vi "write_environment.vi"(9 "Expression":T1, 10 "symbol":string, 11 "Environment in":T3) -> (3 "Environment out":T3)   [LabVIEW 2020]
uses:
  ExpressionType.ctl
  Expression.ctl
  Environment.ctl
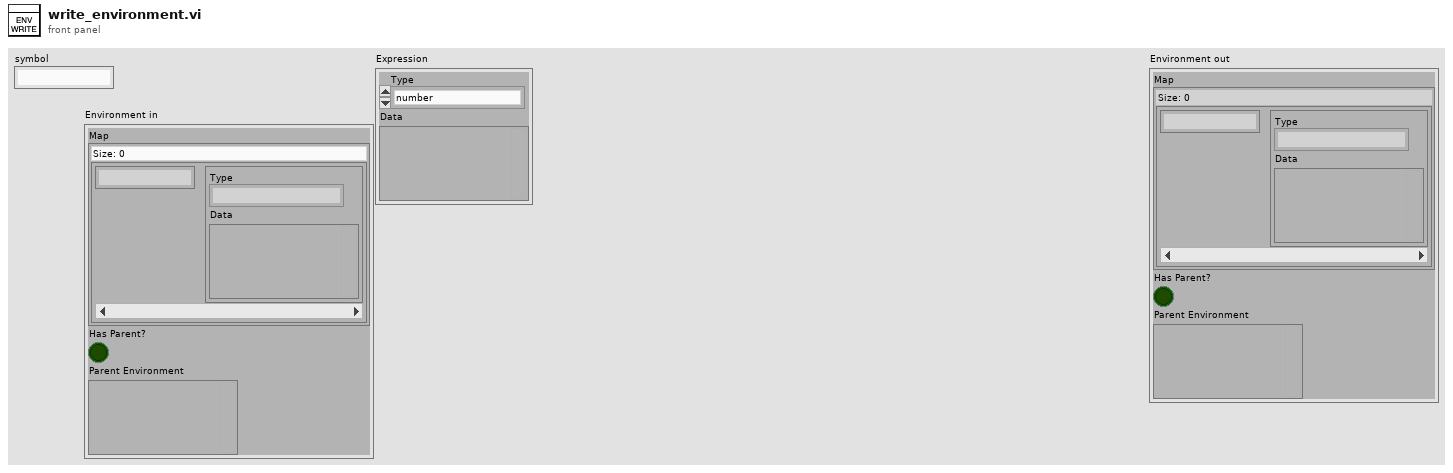
[diagram p1: front panel]
types:
  T1 = typedef "Expression.ctl" = cluster{"Type":T2, "Data":variant}
  T2 = typedef "ExpressionType.ctl" = enum16{"number", "string", "symbol", "primitive", "list", "closure", "macro", "nil", "error"}
  T3 = typedef "Environment.ctl" = cluster{"Map":map{string, T1}, "Has Parent?":bool, "Parent Environment":variant}
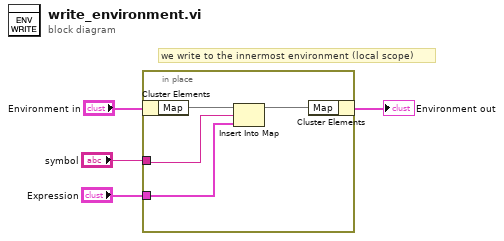
[diagram p0: block diagram]
diagram:
  # "we write to the innermost environment (local scope)"
  n1 = in-place {
    in-place-border: "symbol" -> [w6]
    in-place-border: "Expression" -> [w5]
    n2 = in-place-cluster #1("Environment in") -> ("Map"=w8:map{string, T1})
    n3 = Insert Into Map(map in=w8, key=w6, value=w5) -> (map out=w7:map{string, T1})  [unwired: 2 out]
    n4 = in-place-cluster #1("Map"=w7) -> (→"Environment out":T3)
  }
